vi "StartVideoCapture.vi"(5 "Video Camera":string="USB Camera", 6 "Cycle":i32, 7 "Path to FFMPEG":path=path "C:/Program Files/FFMpeg/bin/ffmpeg.exe", 8 "error in (no error)":errorcluster, 9 "TNom":dbl, 10 "SaveFile":string="DefaultMPegCodec.mp4", 11 "Output Directory":path=path "E:/LTM Tests/VideoTests") -> (0 "error out":errorcluster, 3 "FFMpegProcess":T1)   [LabVIEW 2025]
doc: "Calls FFMPEG to capture and record a video clip.\nVideo clip is stored in sub-directory VIDEOS from Output directory\n\nFilename derived from Cycle count and nominal temperature (TNOM)\nVideo stampedwith timecode, cycle count and nominal temperature"
uses:
  controls/FFMpegRef.ctl
panel:
  in  "SaveType":enum16{"WMV", "MP4"}(ring)=enum."MP4"
  out "command string":string=" -v 8  -f dshow -i video=\"HD Pro Webcam C920\" -fpsmax 20 -vf \"drawtext=fontfile=C\\\\:/Windows/fonts/Arial.ttf :fontsize=36:fontcolor=black:text='%{localtime\\:%y-%m-%d %X.%03N C000 T+000}'\\:box=1:boxborderw=10:x=10:y=H-th-10\"  -y \"E:\\LTM Tests\\VideoTests\\DefaultMPegCodec.mp4.MP4\""
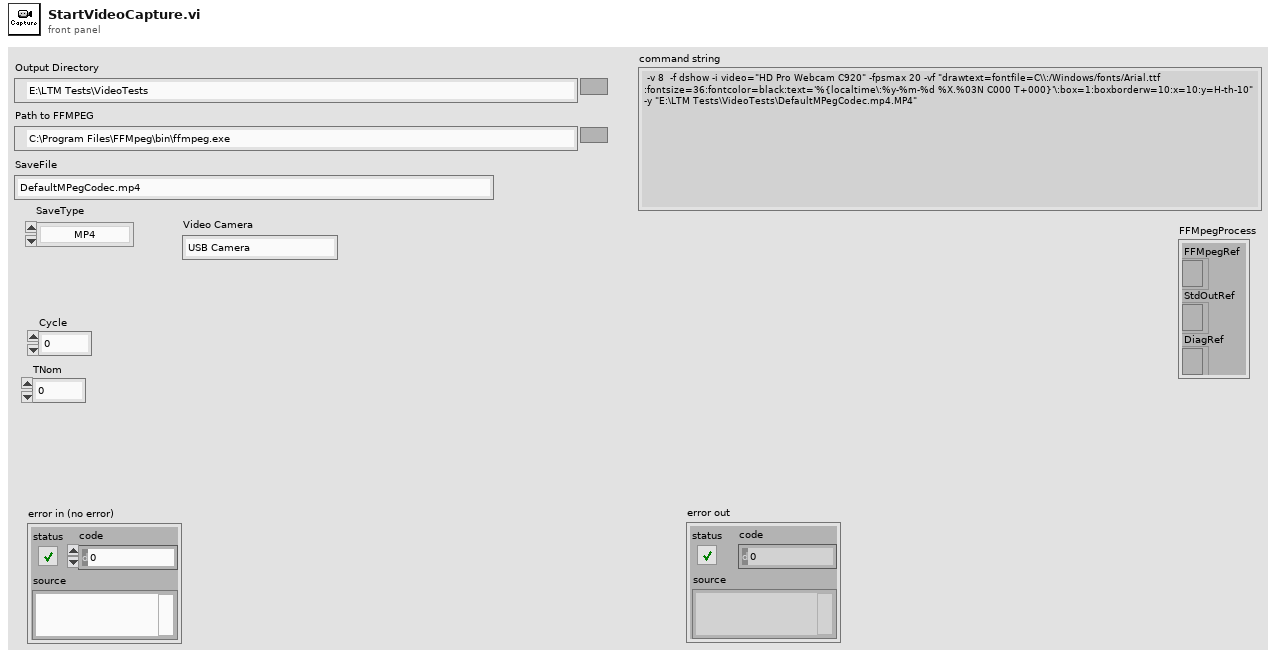
[diagram p1: front panel]
types:
  T1 = typedef "FFMpegRef.ctl" = cluster{"FFMpegRef":refnum<k24>, "StdOutRef":refnum<k24>, "DiagRef":refnum<k24>}
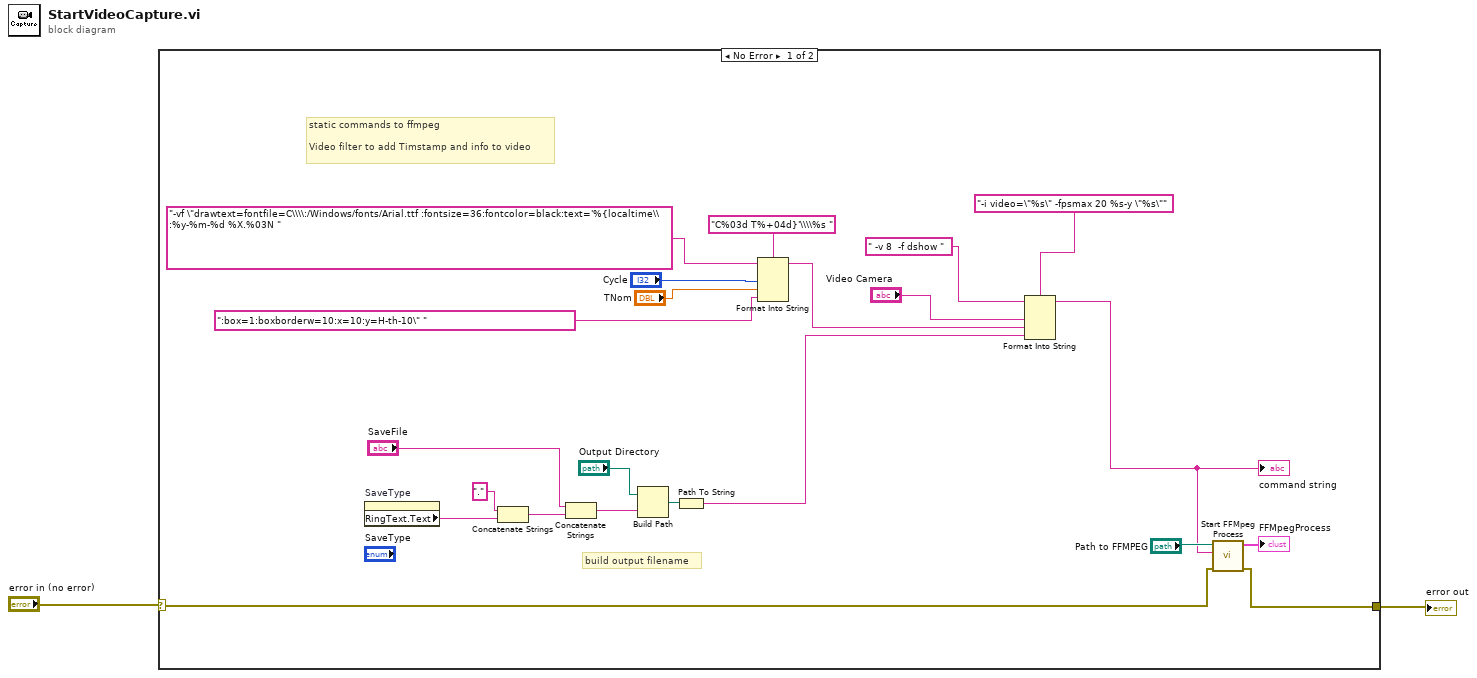
[diagram p0: block diagram]
diagram:
  n1 = case shown="No Error" "error in (no error)" {
    selector: "error in (no error)" -> [w4 w25]
    tunnel: [w3 w25] -> w1
    frame No Error {
      # "build output filename"
      # "static commands to ffmpeg\n\nVideo filter to add Timstamp and info to video"
      n2 = property on="SaveType" class="Enum (strict)"() -> ("RingText.Text"=w19:string)  [unwired: 2 in, 2 out]
      n3 = Concatenate Strings("." ("string"), w19) -> (w18:string)
      n4 = Concatenate Strings("SaveFile", w18) -> (w21:string)
      n5 = Build Path(base path="Output Directory", name or relative path=w21) -> (appended path=w23:path)
      n6 = Path To String(path=w23) -> (string=w8:string)
      n7 = Format Into String(format string="C%03d T%+04d}'\\\\%s ", initial string="-vf \"drawtext=fontfile=C\\\\:/Windows/fonts/Arial.ttf :fontsize=36:fontcolor=black:text='%{localtime\\:%y-%m-%d %X.%03N ", "Cycle", "TNom", ":box=1:boxborderw=10:x=10:y=H-th-10\" ") -> (resulting string=w10:string)  [unwired: 1 in, 1 out]
      n8 = Format Into String(format string="-i video=\"%s\" -fpsmax 20 %s-y \"%s\"", initial string=" -v 8  -f dshow " ("string"), "Video Camera", w10, w8) -> (resulting string=w6:string)  [unwired: 1 in, 1 out]
      "command string" <- w6
      n9 = call "Start FFMpeg Process.vi"("error in (no error)"=w4, "Arguments"=w6, "FFMPEG exe"="Path to FFMPEG") -> ("error out"=w3:errorcluster, "FFMpegProcess"=→"FFMpegProcess":T1)  [unwired: 7 in]
    }
    frame Error {
    }
  }
  "error out" <- w1
